vi "InitSession.vi"(8 "Error Input":errorcluster, 10 "AgentId":string, 11 "LiteAgentSDK Input":refnum<k24>) -> (0 "Error Output":errorcluster, 2 "sessionId":string, 3 "LiteAgentSDK Output":refnum<k24>)   [LabVIEW 2017, in "LiteAgentSDK.lvlib"]
uses:
  LiteAgentSDK.lvlib
  C:/Users/Jan/Projects/LiteAgentSDK-LabVIEW/Source/Bin/LiteAgentSDK.LabVIEW.dll
  Bin/LiteAgentSDK.LabVIEW.dll
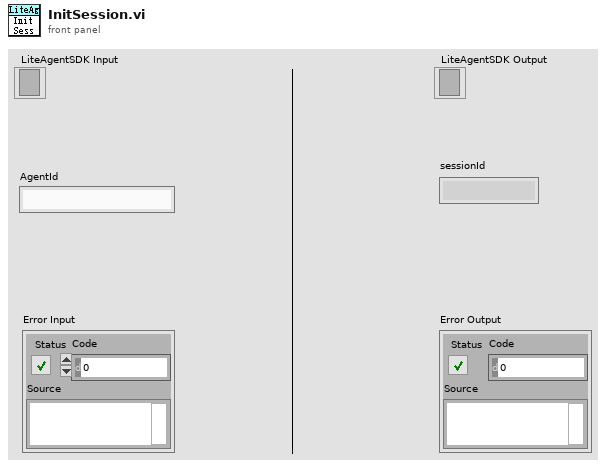
[diagram p1: front panel]
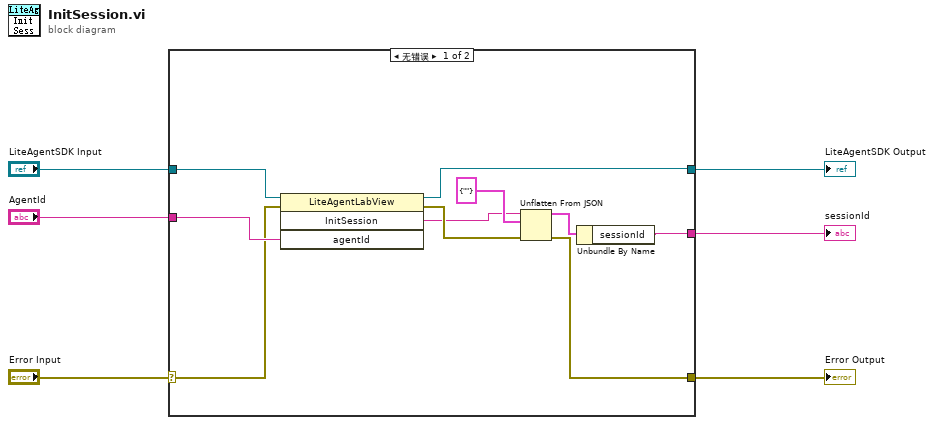
[diagram p0: block diagram]
diagram:
  n1 = case shown="无错误" "Error Input" {
    selector: "Error Input" -> [w12 w17]
    tunnel: "LiteAgentSDK Input" -> [w14 w18]
    tunnel: [w9 w18] -> w2
    tunnel: [w15 w17] -> w5
    tunnel: "AgentId" -> [w13 _]
    tunnel: [w7 _] -> w1
    frame No Error {
      n2 = invoke on="调用节点" class="LiteAgentLabView" method="InitSession"(reference=w14, error in=w12, "agentId"=w13) -> (reference out=w9:refnum<k24>, error out=w11:errorcluster, "InitSession"=w10:string)  [unwired: 1 in, 1 out]
      n3 = Unflatten From JSON(JSON string=w10, type and defaults=cluster{"sessionId":string} {"sessionId"=""} ("Session"), error in (no error)=w11) -> (value=w8:cluster{"sessionId":string}, error out=w15:errorcluster)  [unwired: 4 in]
      n4 = Unbundle By Name(w8) -> ("sessionId"=w7:string)
    }
    frame Error {
    }
  }
  "Error Output" <- w5
  "LiteAgentSDK Output" <- w2
  "sessionId" <- w1
